vi "Manage FPGA Ref FGV.vi"(7 "FPGA Action":T1, 8 "error in":errorcluster, 11 "FPGA resource name":T3) -> (0 "error out":errorcluster, 3 "FPGA Reference Out":T2)   [LabVIEW 2024, in "FPGA Interface.lvlib"]
uses:
  FPGA Interface.lvlib
  <vilib>/userDefined/High Color/nirio_resource_hc.ctl
  Type Definitions/ECU FPGA Reference.ctl
  FPGA Ref Action.ctl
  <vilib>/FPGAPlugInAG/cRIO-9030/niLvFpga_Open_cRIO-9030.vi
  <vilib>/FPGAPlugInAG/cRIO-9030/niLvFpga_Close_cRIO-9030.vi
  <vilib>/rvi/interface/nirviOpenFPGA/nirviOpenFPGA.xnode
  FPGA Bitfiles/ecu-9030_FPGATarget_FPGAMain_pDLqQGhG1UY.lvbitx
  <vilib>/rvi/interface/nirviCloseFPGA/nirviCloseFPGA.xnode
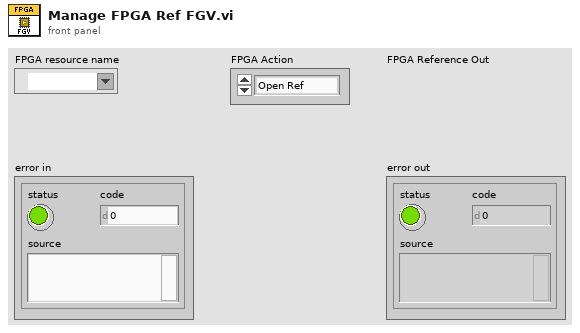
[diagram p1: front panel]
types:
  T1 = typedef "FPGA Interface.lvlib/FPGA Ref Action.ctl" = enum16{"Open Ref", "Get Ref", "Close Ref"}
  T2 = typedef "ECU FPGA Reference.ctl" = refnum<k20>
  T3 = typedef "nirio_resource_hc.ctl" = tag
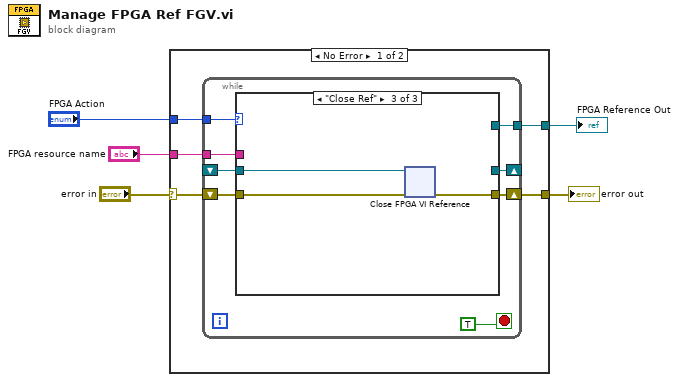
[diagram p0: block diagram]
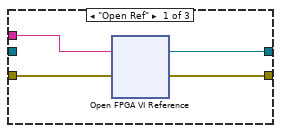
[diagram p2: hidden frame]
diagram:
  n1 = case shown="No Error" "error in" {
    selector: "error in" -> [w6 w28]
    tunnel: "FPGA resource name" -> [w10 _]
    tunnel: [w9 w28] -> w4
    tunnel: "FPGA Action" -> [w8 _]
    tunnel: [w7 _] -> w2
    frame No Error {
      n2 = while {
        tunnel: w10 -> [w17]
        shift-right: [w15] -> w9
        shift-left: w6 -> [w18]
        shift-right: [w16] -> _
        shift-left: _ -> [w12]
        tunnel: w8 -> [w13]
        tunnel: [w11] -> w7
        stop <- TRUE stop-if-true
        n3 = case shown="\"Close Ref\"" w13 {
          tunnel: w18 -> [w22 w23 w25]
          tunnel: w17 -> [w21 _ _]
          tunnel: [w20 w24 _] -> w16
          tunnel: [w19 w23 w27] -> w15
          tunnel: w12 -> [_ w24 w26]
          tunnel: [_ w24 _] -> w11
          frame "Open Ref" {
            n4 = xnode "Open FPGA VI Reference"("error in"=w22, "resource name"=w21) -> ("FPGA VI Reference Out"=w20:T2, "error out"=w19:errorcluster)
          }
          frame "Get Ref", Default {
          }
          frame "Close Ref" {
            n5 = xnode "Close FPGA VI Reference"("FPGA VI Reference In"=w26, "error in"=w25) -> ("error out"=w27:errorcluster)
          }
        }
      }
    }
    frame Error {
    }
  }
  "error out" <- w4
  "FPGA Reference Out" <- w2
